vi "20220107_01.vi"() -> ()   [LabVIEW 2019]
uses:
  <vilib>/numeric/Random Number (Range) DBL.vi
panel:
  in  "Stop":bool
  out "element":dbl
  in  "Flush":bool
  out "enque timed out?":bool
  out "elements":dbl[](array[numeric])
  in  "Lossy Enque":bool
  in  "Enque":bool
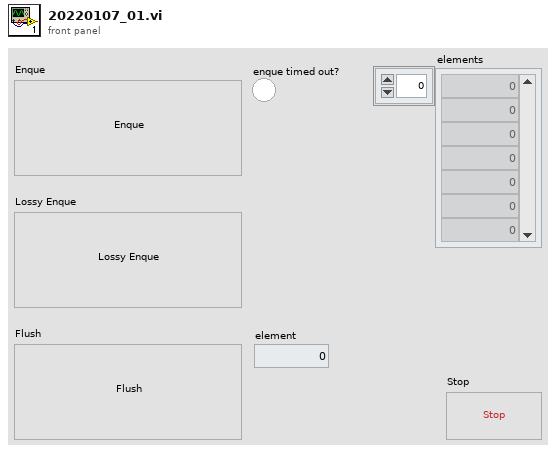
[diagram p1: front panel]
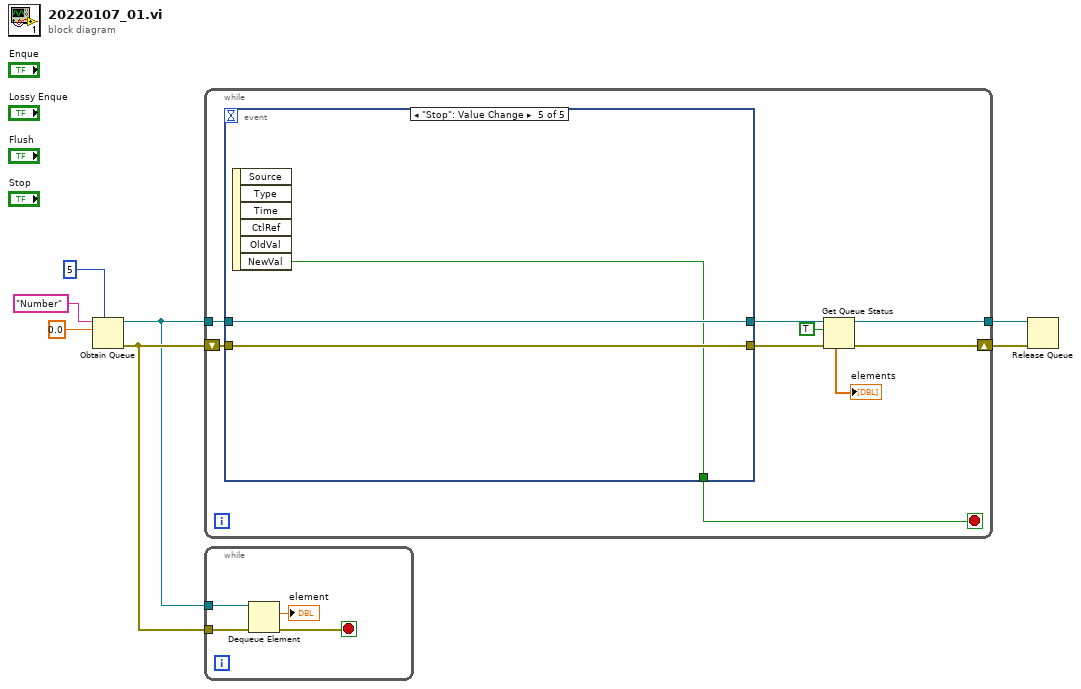
[diagram p0: block diagram]
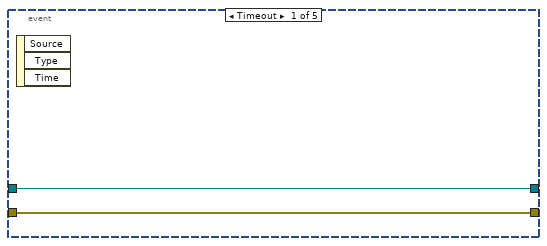
[diagram p2: hidden frame]
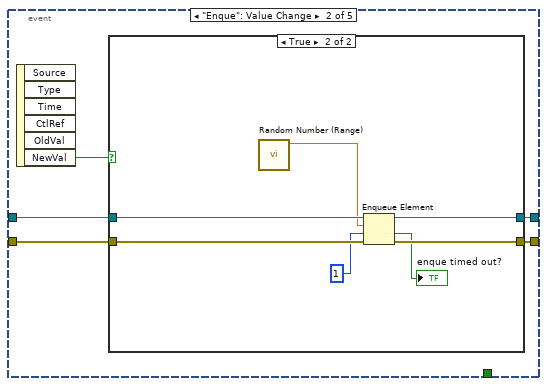
[diagram p3: hidden frame]
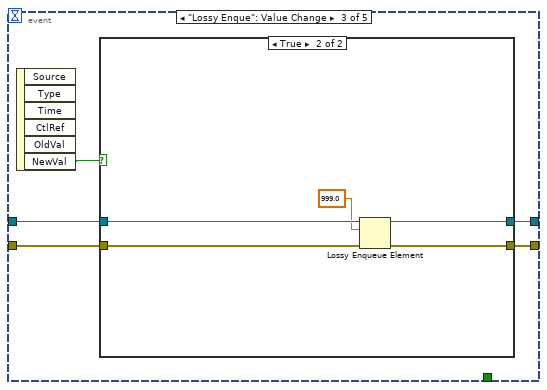
[diagram p5: hidden frame]
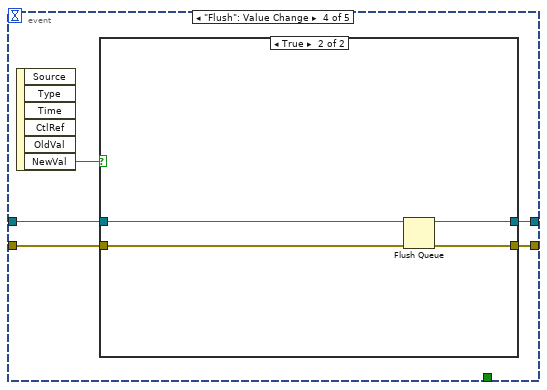
[diagram p7: hidden frame]
diagram:
  n1 = Obtain Queue(max queue size (-1, unlimited)=5, name (unnamed)="Number", element data type=0.0) -> (queue out=w1:refnum<queue>, error out=w2:errorcluster)  [unwired: 2 in, 1 out]
  n2 = while {
    shift-right: [w12] -> w5
    shift-left: w2 -> [w15]
    tunnel: w1 -> [w16]
    tunnel: [w11] -> w4
    stop <- w8 stop-if-true
    n3 = event shown="[4] \"Stop\": Value Change" {
      selector: _ -> [_ _ _ _ _]
      dyn-events: _ -> [_ _ _ _ _]
      timeout: _ -> [_ _ _ _ _]
      tunnel: w16 -> [w17 w22 w35 w47 w57]
      tunnel: w15 -> [w18 w21 w36 w48 w58]
      tunnel: [w18 w20 w34 w46 w58] -> w14
      tunnel: [w17 w19 w33 w45 w57] -> w13
      tunnel: [_ _ _ _ w56] -> w8
      event Timeout {
        n4 = event-data() -> ()  [unwired: 1 in, 3 out]
      }
      event "Enque": Value Change {
        n5 = event-data() -> ("NewVal"=w23:bool)  [unwired: 1 in, 5 out]
        n6 = case shown="True" w23 {
          tunnel: w22 -> [w24 w32]
          tunnel: w21 -> [w25 w31]
          tunnel: [w25 w30] -> w20
          tunnel: [w24 w29] -> w19
          frame False {
          }
          frame True {
            n7 = call-poly <vilib>:"Random Number (Range).vi"() -> ("number"=w28:dbl)  [unwired: 11 in]
            n8 = Enqueue Element(queue=w32, element=w28, timeout in ms (-1)=1, error in (no error)=w31) -> (queue out=w29:refnum<queue>, timed out?=→"enque timed out?":bool, error out=w30:errorcluster)
          }
        }
      }
      event "Lossy Enque": Value Change {
        n9 = event-data() -> ("NewVal"=w37:bool)  [unwired: 1 in, 5 out]
        n10 = case shown="True" w37 {
          tunnel: w36 -> [w39 w44]
          tunnel: w35 -> [w38 w43]
          tunnel: [w39 w42] -> w34
          tunnel: [w38 w41] -> w33
          frame False {
          }
          frame True {
            n11 = Lossy Enqueue Element(queue=w43, element=999.0, error in (no error)=w44) -> (queue out=w41:refnum<queue>, error out=w42:errorcluster)  [unwired: 2 out]
          }
        }
      }
      event "Flush": Value Change {
        n12 = event-data() -> ("NewVal"=w49:bool)  [unwired: 1 in, 5 out]
        n13 = case shown="True" w49 {
          tunnel: w48 -> [w51 w55]
          tunnel: w47 -> [w50 w52]
          tunnel: [w51 w54] -> w46
          tunnel: [w50 w53] -> w45
          frame False {
          }
          frame True {
            n14 = Flush Queue(queue=w52, error in (no error)=w55) -> (queue out=w53:refnum<queue>, error out=w54:errorcluster)  [unwired: 1 out]
          }
        }
      }
      event "Stop": Value Change {
        n15 = event-data() -> ("NewVal"=w56:bool)  [unwired: 1 in, 5 out]
      }
    }
    n16 = Get Queue Status(queue=w13, return elements? (F)=TRUE, error in (no error)=w14) -> (queue out=w11:refnum<queue>, error out=w12:errorcluster, elements=→"elements":dbl[])  [unwired: 5 out]
  }
  n17 = while {
    tunnel: w2 -> [w62]
    tunnel: w1 -> [w61]
    stop <- w59 stop-if-true
    n18 = Dequeue Element(queue=w61, error in (no error)=w62) -> (element=→"element":dbl, error out=w59:errorcluster)  [unwired: 1 in, 2 out]
  }
  n19 = Release Queue(queue=w4, error in (no error)=w5) -> ()  [unwired: 1 in, 3 out]
